vi "getXMLNodeFromTop.vi"(8 "error in (no error)":errorcluster, 11 "xmlNode in":refnum<class "xmlNode.lvclass">) -> (0 "error out":errorcluster, 2 "xmlNode exracted":refnum<class "xmlNode.lvclass">, 3 "xmlNode out":refnum<class "xmlNode.lvclass">)   [LabVIEW 2009, in "Tools.lvlib" / "xml.lvlib" / "xmlNode.lvclass"]
uses:
  xmlNode.lvclass
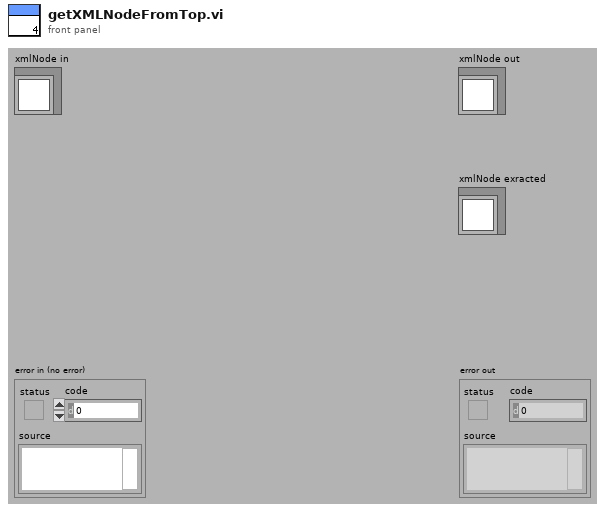
[diagram p1: front panel]
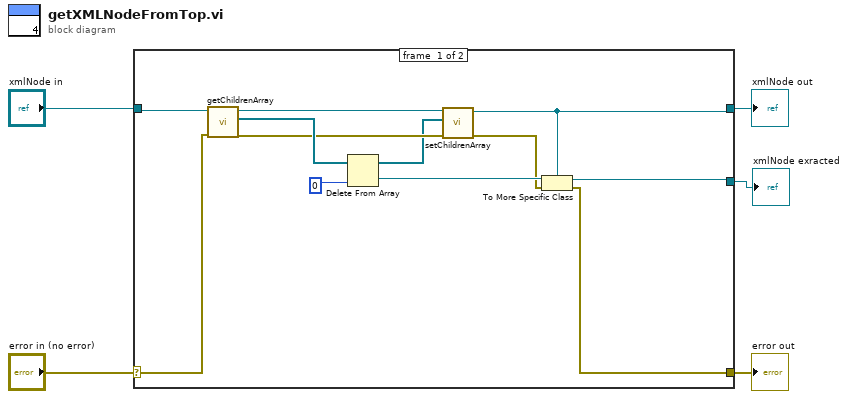
[diagram p0: block diagram]
diagram:
  n1 = case shown="No Error" "error in (no error)" {
    selector: "error in (no error)" -> [w16 w19]
    tunnel: [w8 w19] -> w4
    tunnel: [w12 w18] -> w2
    tunnel: "xmlNode in" -> [w17 w18]
    tunnel: [w11 _] -> w1
    frame #0 {
      n2 = call-dynamic "getChildrenArray.vi"("error in (no error)"=w16, "xmlNode.lvclass in"=w17) -> ("error out"=w13:errorcluster, "Children"=w15:refnum<class "xmlNode.lvclass">[], "xmlNode.lvclass out"=w14:refnum<class "xmlNode.lvclass">)  [unwired: 7 in]
      n3 = Delete From Array(array=w15, index=0) -> (deleted portion=w9:refnum<class "xmlNode.lvclass">, array with subset deleted=w10:refnum<class "xmlNode.lvclass">[])  [unwired: 1 in]
      n4 = call-dynamic "setChildrenArray.vi"("error in (no error)"=w13, "Children"=w10, "xmlNode.lvclass in"=w14) -> ("error out"=w7:errorcluster, "xmlNode.lvclass out"=w12:refnum<class "xmlNode.lvclass">)  [unwired: 7 in]
      n5 = To More Specific Class(target class=w12, reference=w9, error in=w7) -> (specific class reference=w11:refnum<class "xmlNode.lvclass">, error out=w8:errorcluster)
    }
    frame #1 {
    }
  }
  "error out" <- w4
  "xmlNode out" <- w2
  "xmlNode exracted" <- w1
